vi "TDMS Get Number of Groups.vi"(8 "error in (no error)":errorcluster, 11 "path":path) -> (0 "error out":errorcluster, 2 "# of groups":i32)   [LabVIEW 2016]
panel:
  out "file path out":path
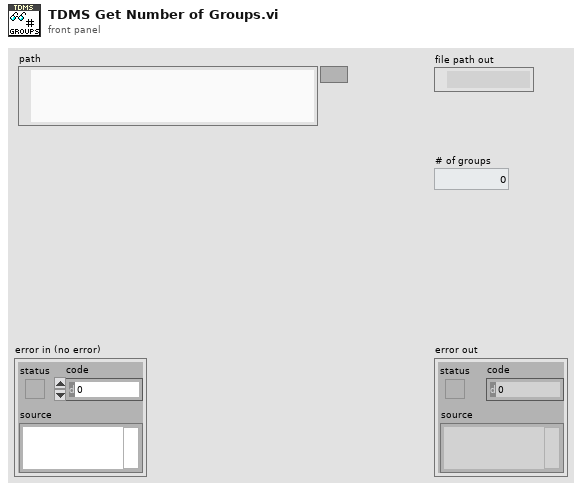
[diagram p1: front panel]
types:
  T1 = enum16{"open", "open or create", "create or replace", "create", "open (read-only)"}
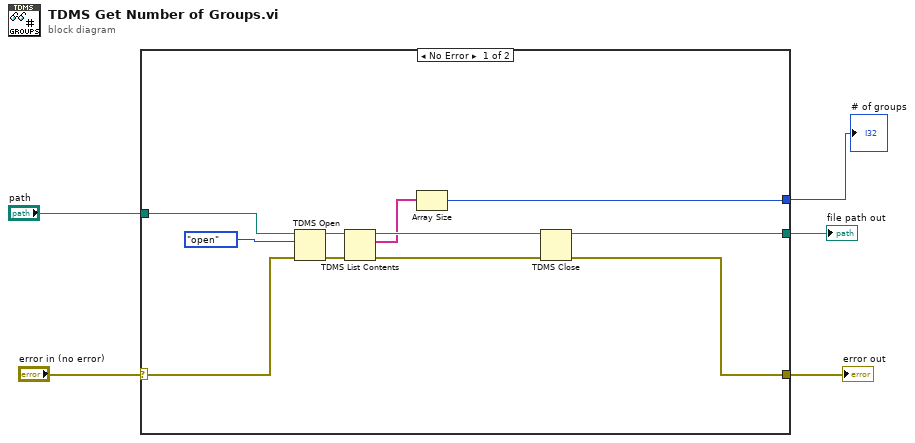
[diagram p0: block diagram]
diagram:
  n1 = case shown="No Error" "error in (no error)" {
    selector: "error in (no error)" -> [w13 w17]
    tunnel: [w15 w17] -> w4
    tunnel: "path" -> [w14 _]
    tunnel: [w12 _] -> w2
    tunnel: [w6 _] -> w1
    frame No Error {
      n2 = TDMS Open(8:w13, 10:T1."open" ("operation (0:open)"), 11:w14) -> (0:w10:errorcluster, 3:w11:refnum<k34>)  [unwired: 4 in]
      n3 = TDMS List Contents(4:w10, 7:w11) -> (0:w9:errorcluster, 2:w7:string[], 3:w8:refnum<k34>)  [unwired: 1 in, 1 out]
      n4 = Array Size(array=w7) -> (size(s)=w6:i32)
      n5 = TDMS Close(8:w9, 11:w8) -> (0:w15:errorcluster, 3:w12:path)
    }
    frame Error {
    }
  }
  "error out" <- w4
  "file path out" <- w2
  "# of groups" <- w1
